vi "Teleop.vi"(10 "Match Info":T1={"Autonomous Elapsed Seconds"=0.0, "TeleOp Elapsed Seconds"=0.0, "Disabled Elapsed Seconds"=0.0, "Visited Autonomous"=FALSE, "Visited TeleOp"=FALSE, "Visited Disabled"=FALSE, "Autonomous Settings"={"Autonomous Style"=enum."Independent", "VI Refnum"=refnum}}, 11 "Call Context":T2) -> ()   [LabVIEW 2012]
doc: "This VI is called for each TeleOp packet received from the DS where the robot is not disabled. It is often used to read from the joysticks and update I/O or to update setpoints for timed control loops. It should complete and return within 20 milliseconds or it may miss DS packets."
uses:
  <vilib>/Rock Robotics/WPI/DriverStation/WPI_DriverStationDerivedRobotMode.ctl
  <vilib>/Rock Robotics/WPI/DriverStation/WPI_DriverStationMatch Info.ctl
  Robot Global Data.vi
  <vilib>/Rock Robotics/WPI/Joystick/WPI_JoystickGetSetRefNum.vi
  <vilib>/Rock Robotics/WPI/RobotDrive/WPI_RobotDriveGetSetRefNum.vi
panel:
  out "Numeric 1":dbl(slide) scale=0.0..100.0
  out "Boolean 2":bool
  out "Boolean 1":bool
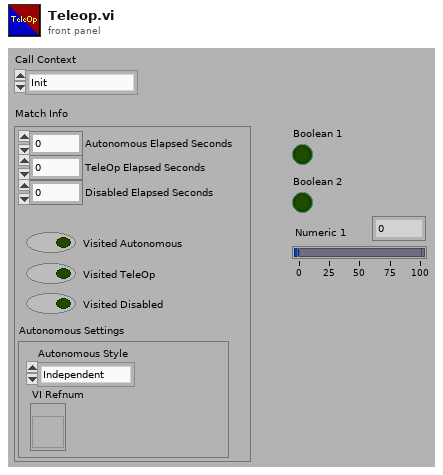
[diagram p1: front panel]
types:
  T1 = typedef "WPI_DriverStationMatch Info.ctl" = cluster{"Autonomous Elapsed Seconds":dbl, "TeleOp Elapsed Seconds":dbl, "Disabled Elapsed Seconds":dbl, "Visited Autonomous":bool, "Visited TeleOp":bool, "Visited Disabled":bool, "Autonomous Settings":cluster{"Autonomous Style":enum16{"Iterative", "Independent"}, "VI Refnum":refnum<vi>}}
  T2 = typedef "WPI_DriverStationDerivedRobotMode.ctl" = enum16{"Init", "Execute", "Stop"}
  T3 = typedef "WPI_JoystickDevRef.ctl" = cluster{"Device":T4}
  T4 = typedef "WPI_JoystickDeviceEnum.ctl" = enum16{"USB 1", "USB 2", "USB 3", "USB 4", "Kinect 1", "Kinect 2"}
  T5 = typedef "WPI_JoystickButtonState.ctl" = cluster{"Button 1":bool, "Button 2":bool, "Button 3":bool, "Button 4":bool, "Button 5":bool, "Button 6":bool, "Button 7":bool, "Button 8":bool, "Button 9":bool, "Button 10":bool, "Button 11":bool, "Button 12":bool}
  T6 = cluster{"axis 1 (x)":dbl, "axis 2 (y)":dbl, "axis 3 (throttle)":dbl, "axis 4":dbl, "axis 5":dbl, "axis 6":dbl}
  T7 = enum16{"Off", "2pt Key Shot", "3pt Key Shot", "Back Shot", "Fender Shot"}
  T8 = typedef "WPI_RobotDriveDevRef.ctl" = cluster{"DevStatus":errorcluster, "Motors[]":T9[], "Square Inputs":bool, "Max Output":dbl, "Isochronous":bool}
  T9 = typedef "WPI_MotorControlDeviceRef.ctl" = cluster{"DeviceStatus":errorcluster, "Type":enum16{"PWM", "CAN"}, "PWM":cluster{"Digital Module":T10, "PWM Channel":T11, "DeadBand":T12}, "CAN":cluster{"Device Number":u8, "Control Mode":T13, "Semaphore":T14, "Max Vout":dbl}, "Invert":bool, "TransformRef":T15, "InvTransformRef":T15}
  T10 = typedef "FPGA_TypedefDigitalModule.ctl" = enum16{"Digital Module 1", "Digital Module 2"}
  T11 = typedef "FPGA_DIOPWMChannel.ctl" = enum8{"PWM 1", "PWM 2", "PWM 3", "PWM 4", "PWM 5", "PWM 6", "PWM 7", "PWM 8", "PWM 9", "PWM 10", "Invalid"}
  T12 = typedef "WPI_PWMDeadband.ctl" = cluster{"Name":string, "maxPositivePwm":i32, "minPositivePwm":i32, "centerPwm":i32, "maxNegativePwm":i32, "minNegativePwm":i32, "angularRange":u16}
  T13 = typedef "WPI_CANJaguar_ControlMode.ctl" = enum8{"Percent VBus", "Current", "Speed", "Position", "Voltage"}
  T14 = typedef "Semaphore RefNum" = refnum<k1>
  T15 = typedef "WPI_PWMTransform_ConPane.ctl" = refnum<vi>
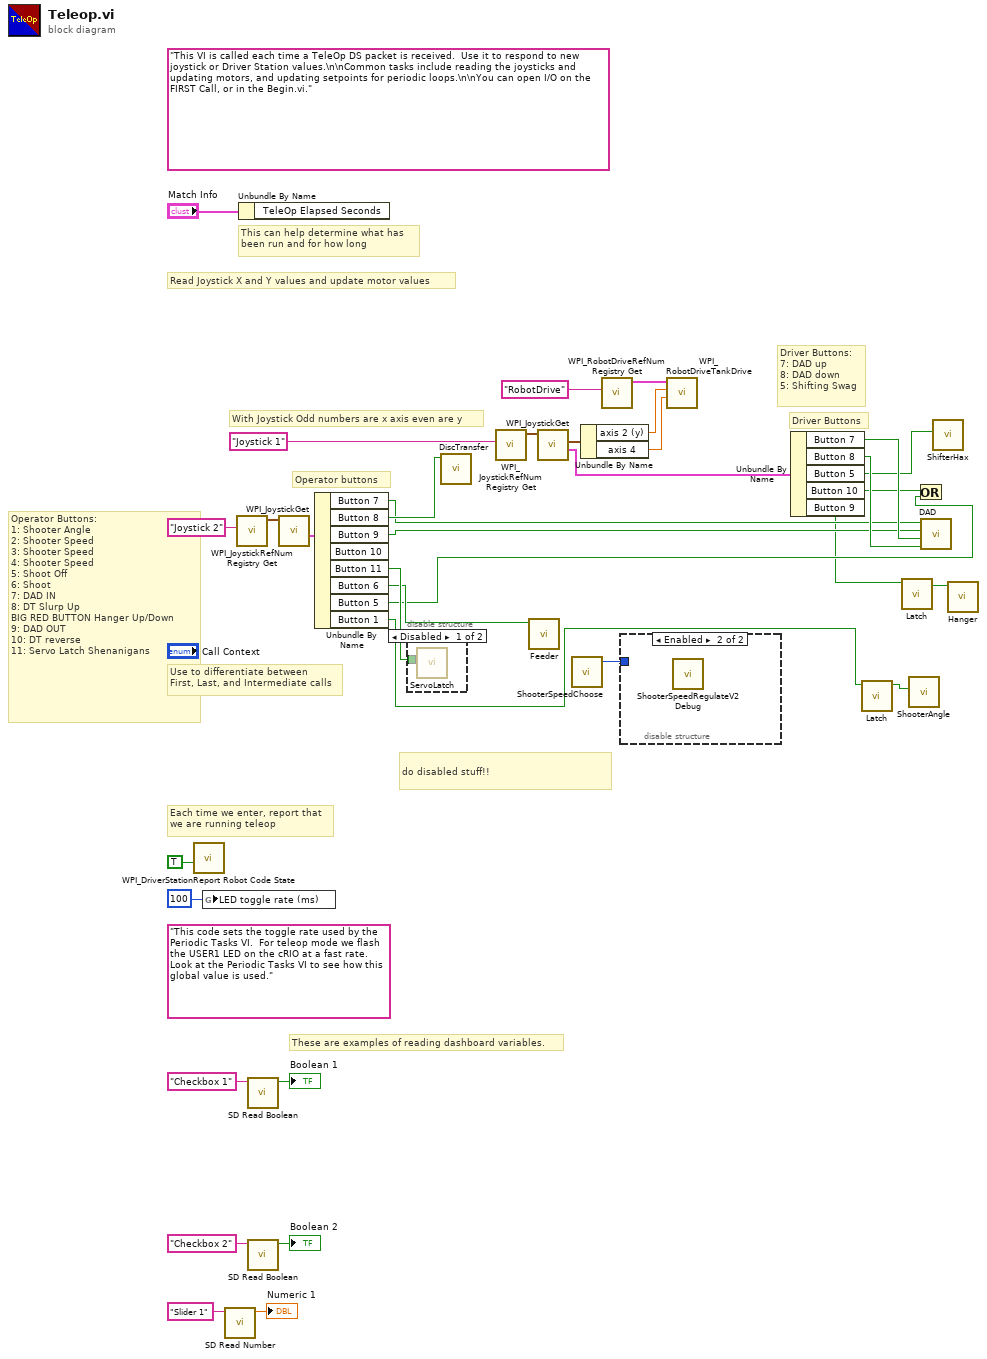
[diagram p0: block diagram]
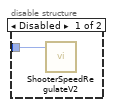
[diagram p3: hidden frame]
diagram:
  (unwired) "This code sets the toggle rate used by the Periodic Tasks VI.  For teleop mode we flash the USER1 LED on the cRIO at a fast rate.  Look at the Periodic Tasks VI to see how this global value is used."
  (unwired) "This VI is called each time a TeleOp DS packet is received.  Use it to respond to new joystick or Driver Station values.\n\nCommon tasks include reading the joysticks and updating motors, and updating setpoints for periodic loops.\n\nYou can open I/O on the FIRST Call, or in the Begin.vi."
  # "do disabled stuff!!"
  # "Driver Buttons:\n7: DAD up\n8: DAD down \n5: Shifting Swag"
  # "Operator Buttons:\n1: Shooter Angle\n2: Shooter Speed\n3: Shooter Speed\n4: Shooter Speed\n5: Shoot Off\n6: Shoot\n7: DAD IN\n8: DT Slurp Up \nBIG RED BUTTON Hanger Up/Down\n9: DAD OUT\n10: DT reverse \n11: Servo Latch Shenanigans"
  # "Driver Buttons"
  # "Operator buttons"
  # "With Joystick Odd numbers are x axis even are y"
  # "These are examples of reading dashboard variables."
  # "Each time we enter, report that\nwe are running teleop"
  # "Use to differentiate between\nFirst, Last, and Intermediate calls"
  # "This can help determine what has\nbeen run and for how long"
  # "Read Joystick X and Y values and update motor values"
  n1 = call <vilib>:"WPI_DriverStationReport Robot Code State.vi"("TeleOp"=TRUE ("Autonomous")) -> ()  [unwired: 10 in, 1 out]
  n2 = global write "Robot Global Data.vi" "LED toggle rate (ms)"(u32 100 ("LED ms toggle rate")) -> ()
  n3 = call <vilib>:"SD Read Number.vi"("Name"="Slider 1" ("refnum name")) -> ("Numeric"=→"Numeric 1":dbl)  [unwired: 8 in, 2 out]
  n4 = call <vilib>:"WPI_JoystickRefNum Registry Get.vi"("refnum name"="Joystick 2") -> ("JoystickDevRef"=w21:T3)  [unwired: 1 in, 9 out]
  n5 = Unbundle By Name("Match Info") -> ()  [unwired: 1 out]
  n6 = call <vilib>:"SD Read Boolean.vi"("Name"="Checkbox 1" ("refnum name")) -> ("Boolean"=→"Boolean 1":bool)  [unwired: 8 in, 2 out]
  n7 = call <vilib>:"SD Read Boolean.vi"("Name"="Checkbox 2" ("refnum name")) -> ("Boolean"=→"Boolean 2":bool)  [unwired: 8 in, 2 out]
  n8 = call <vilib>:"WPI_JoystickGet.vi"("JoystickDevRef"=w21) -> ("Buttons"=w19:T5)  [unwired: 1 in, 5 out]
  n9 = Unbundle By Name(w19) -> ("Button 7"=w3:bool, "Button 8"=w4:bool, "Button 9"=w2:bool, "Button 11"=w12:bool, "Button 6"=w11:bool, "Button 5"=w6:bool, "Button 1"=w5:bool)  [unwired: 1 out]
  n10 = disable-structure shown="Disabled" {
    disable-tunnel: w12 -> [w36 _]
    frame Disabled {
      n11 = call "ServoLatch.vi"("Button X Hit"=w36) -> ()  [unwired: 11 in]
    }
    frame Enabled {
    }
  }
  n12 = call "DiscTransfer.vi"("DT Foward Button"=w4) -> ()  [unwired: 11 in]
  n13 = call <vilib>:"WPI_JoystickRefNum Registry Get.vi"("refnum name"="Joystick 1") -> ("JoystickDevRef"=w32:T3)  [unwired: 1 in, 9 out]
  n14 = call "Feeder.vi"("SHOOT Button"=w11) -> ()  [unwired: 10 in, 1 out]
  n15 = call <vilib>:"WPI_JoystickGet.vi"("JoystickDevRef"=w32) -> ("Buttons"=w22:T5, "Axes"=w29:T6)  [unwired: 1 in, 4 out]
  n16 = call "ShooterSpeedChoose.vi"() -> ("Shooter Speed"=w10:T7)  [unwired: 11 in]
  n17 = Unbundle By Name(w29) -> ("axis 2 (y)"=w17:dbl, "axis 4"=w16:dbl)
  n18 = call <vilib>:"WPI_RobotDriveRefNum Registry Get.vi"("refnum name"="RobotDrive") -> ("RobotDriveDevRef"=w23:T8)  [unwired: 1 in, 9 out]
  n19 = disable-structure shown="Enabled" {
    disable-tunnel: w10 -> [w37 _]
    frame Disabled {
      n20 = call "ShooterSpeedRegulateV2.vi"("Shooter Speed"=w37) -> ()  [unwired: 13 in, 2 out]
    }
    frame Enabled {
      n21 = call "ShooterSpeedRegulateV2 Debug.vi"() -> ()  [unwired: 14 in, 2 out]
    }
  }
  n22 = call <vilib>:"WPI_RobotDriveTankDrive.vi"("Right axis value"=w16, "Left axis value"=w17, "RobotDriveDevRef"=w23) -> ()  [unwired: 6 in, 3 out]
  n23 = Unbundle By Name(w22) -> ("Button 7"=w14:bool, "Button 8"=w15:bool, "Button 5"=w13:bool, "Button 10"=w7:bool, "Button 9"=w1:bool)
  n24 = call "Latch.vi"("Latch In"=w5) -> ("Latch Out"=w8:bool)  [unwired: 10 in]
  n25 = call "Latch.vi"("Latch In"=w1) -> ("Latch Out"=w9:bool)  [unwired: 10 in]
  n26 = call "ShooterAngle.vi"("Shooter Angle Up?"=w8) -> ()  [unwired: 11 in]
  n27 = Or(x=w7, y=w6) -> ()  [unwired: 1 out]
  n28 = call "DAD.vi"("BAD DOWN"=w15, "BAD UP"=w14, "BAD OUT"=w2, "BAD IN"=w3) -> ()  [unwired: 7 in, 1 out]
  n29 = call "ShifterHax.vi"("Shifter Button"=w13) -> ()  [unwired: 11 in]
  n30 = call "Hanger.vi"("Hanger Up"=w9) -> ()  [unwired: 10 in, 1 out]
